vi "Create Directory.vi"(0 "directory":path, 11 "error in":errorcluster) -> (4 "dup directory":path, 15 "error out":errorcluster)   [LabVIEW 2021, in "Path Functions.lvlib"]
uses:
  Path Functions.lvlib
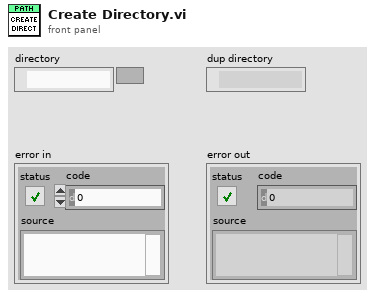
[diagram p1: front panel]
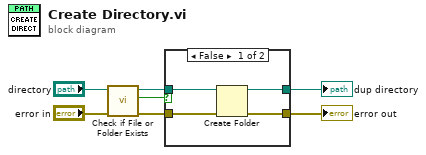
[diagram p0: block diagram]
diagram:
  n1 = call <vilib>:"Check if File or Folder Exists.vi"("error in (no error)"="error in", "path"="directory") -> ("error out"=w4:errorcluster, "file or folder exists?"=w5:bool, "dup path"=w6:path)  [unwired: 7 in]
  n2 = case shown="False" w5 {
    tunnel: w4 -> [w11 w13]
    tunnel: [w10 w13] -> w2
    tunnel: [w8 w12] -> w1
    tunnel: w6 -> [w9 w12]
    frame False {
      n3 = Create Folder(path (use dialog)=w9, error in=w11) -> (created path=w8:path, error out=w10:errorcluster)  [unwired: 1 in, 1 out]
    }
    frame True {
    }
  }
  "error out" <- w2
  "dup directory" <- w1
